vi "Read Direction.vi"(8 "error in (no error)":errorcluster, 11 "Image Gallery.lvclass in":refnum<class "Image Gallery.lvclass">) -> (0 "error out":errorcluster, 2 "Direction":enum16{"Forward", "Backward"}(ring), 3 "Image Gallery.lvclass out":refnum<class "Image Gallery.lvclass">)   [LabVIEW 2012, in "ImageGallery.lvlib" / "Image Gallery.lvclass"]
uses:
  Image Gallery.lvclass
  Image Gallery.lvclass/Image Gallery.ctl
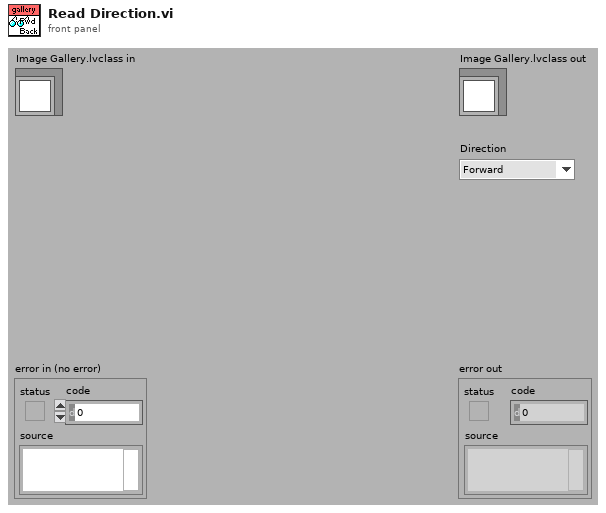
[diagram p1: front panel]
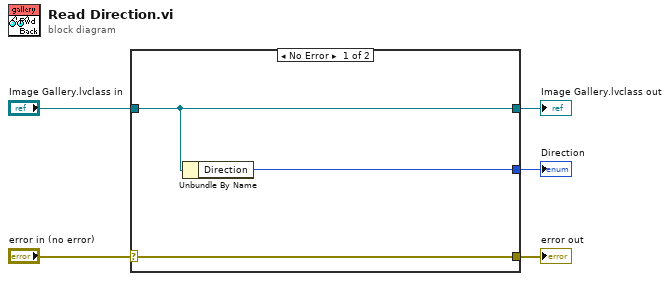
[diagram p0: block diagram]
diagram:
  n1 = case shown="No Error" "error in (no error)" {
    selector: "error in (no error)" -> [w8 w9]
    tunnel: [w8 w9] -> w4
    tunnel: [w7 w10] -> w2
    tunnel: "Image Gallery.lvclass in" -> [w7 w10]
    tunnel: [w6 _] -> w1
    frame No Error {
      n2 = Unbundle By Name(w7) -> ("Direction"=w6:enum16{"Forward", "Backward"})
    }
    frame Error {
    }
  }
  "error out" <- w4
  "Image Gallery.lvclass out" <- w2
  "Direction" <- w1
